vi "FTW-Crypto-PublicKeySignature-GenerateKeys.vi"(0 "KeySize [384, 16384]":i32=1024, 11 "error in":errorcluster) -> (4 "Private Key":string, 6 "Public Key":string, 8 "Abbreviated Public Key":string, 15 "error out":errorcluster)   [LabVIEW 2012]
uses:
  <vilib>/regexp/Match Regular Expression_ExecuteOffsets.vi
panel:
  # "Inputs"
  # "Outputs"
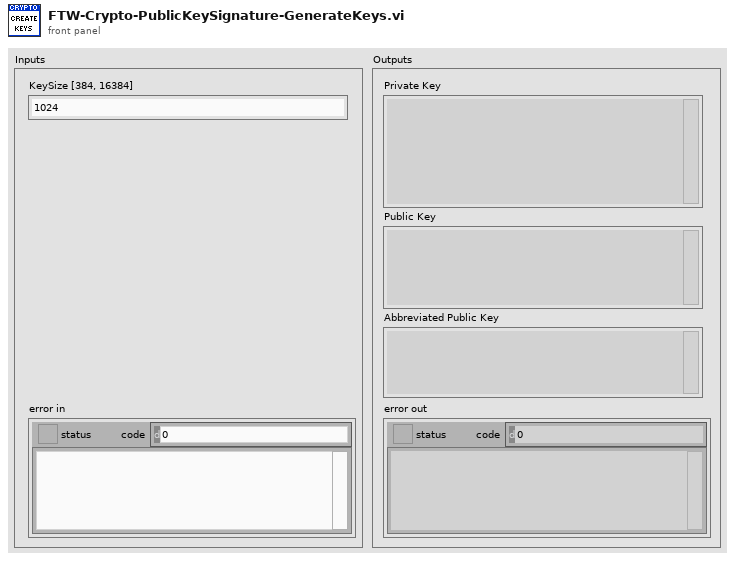
[diagram p1: front panel]
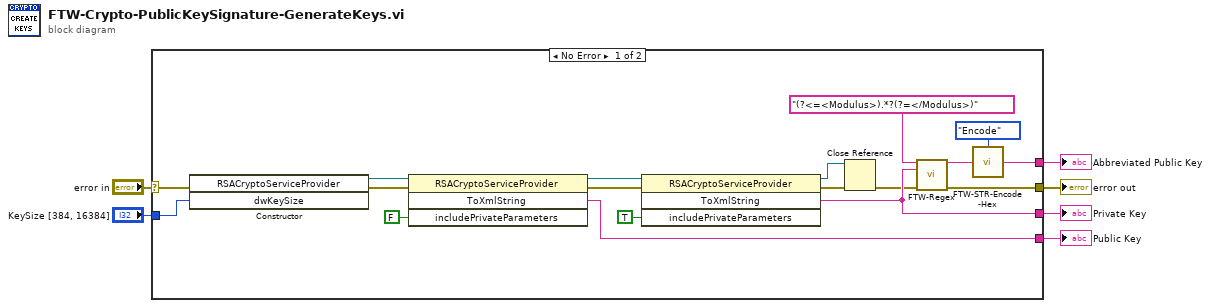
[diagram p0: block diagram]
diagram:
  n1 = case shown="No Error" "error in" {
    selector: "error in" -> [w20 w25]
    tunnel: [w14 w25] -> w5
    tunnel: "KeySize [384, 16384]" -> [w21 _]
    tunnel: [w17 _] -> w3
    tunnel: [w16 _] -> w2
    tunnel: [w8 _] -> w1
    frame No Error {
      n2 = constructor class="RSACryptoServiceProvider"(error in=w20, "dwKeySize"=w21) -> (reference out=w9:refnum<k24>, error out=w12:errorcluster)  [unwired: 2 in, 2 out]
      n3 = invoke class="RSACryptoServiceProvider" method="ToXmlString"(reference=w9, error in=w12, "includePrivateParameters"=FALSE) -> (reference out=w10:refnum<k24>, error out=w11:errorcluster, "ToXmlString"=w8:string)  [unwired: 1 in, 1 out]
      n4 = invoke class="RSACryptoServiceProvider" method="ToXmlString"(reference=w10, error in=w11, "includePrivateParameters"=TRUE) -> (reference out=w19:refnum<k24>, error out=w18:errorcluster, "ToXmlString"=w16:string)  [unwired: 1 in, 1 out]
      n5 = Close Reference(reference=w19, error in (no error)=w18) -> (error out=w15:errorcluster)
      n6 = call "FTW-Regex.vi"("Regular Expression"="(?<=<Modulus>).*?(?=</Modulus>)" ("Input String"), "Input String"=w16, "error in"=w15) -> ("Match"=w23:string, "error out"=w14:errorcluster)  [unwired: 8 in, 3 out]
      n7 = call "FTW-STR-Encode-Hex.vi"("Input"=w23, "Direction"=enum16{"Encode", "Decode"}."Encode") -> ("Output"=w17:string)
    }
    frame Error {
    }
  }
  "Private Key" <- w2
  "error out" <- w5
  "Abbreviated Public Key" <- w3
  "Public Key" <- w1
